vi "Start.vi"(6 "Teller":T1 {"Absolute Time" format="%<%x %.3X>T"}, 8 "Error in":errorcluster, 11 "Start jettl Msg in":refnum<class "Start jettl Msg.lvclass">) -> (0 "Error out":errorcluster, 3 "Start jettl Msg out":refnum<class "Start jettl Msg.lvclass">)   [LabVIEW 2020, in "jettl.lvlib" / "Start jettl Msg.lvlib" / "Start jettl Msg.lvclass"]
doc: "jettl 6.14.1.98\nNathan Davis - Nathan Davis\nCopyright (c) 2026, Nathan Davis\nMIT"
uses:
  Start jettl Msg.lvclass
  Teller Metadata/Teller Metadata.lvclass
  Relation.ctl
  jettl.lvlib
  Teller.ctl
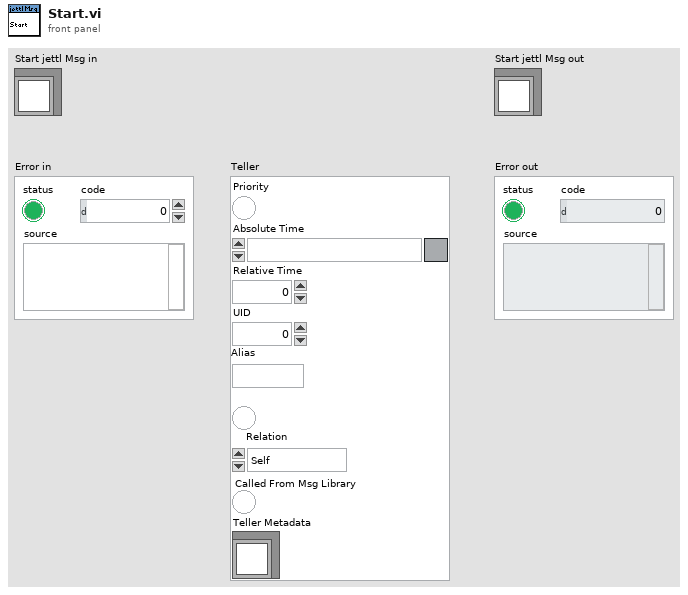
[diagram p1: front panel]
types:
  T1 = typedef "jettl.lvlib/Teller.ctl" = cluster{"Priority":bool, "Absolute Time":timestamp, "Relative Time":dbl, "UID":i32, "Alias":string, "Valid Relation":bool, "Relation":T2, "Called From Msg Library":bool, "Teller Metadata":refnum<class "Teller Metadata.lvclass">}
  T2 = typedef "jettl.lvlib/Relation.ctl" = enum16{"Self", "Parent", "Child"}
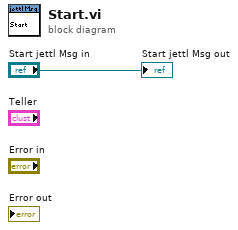
[diagram p0: block diagram]
diagram:
  "Start jettl Msg out" <- "Start jettl Msg in"
